vi "Exercise1.3-Accumulator_For.vi"() -> ()   [LabVIEW 2013]
panel:
  out "Array":i32[](array[numeric])
  out "Sum":i32
  in  "N":i32
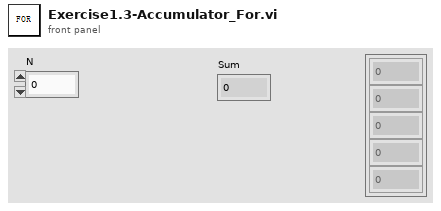
[diagram p1: front panel]
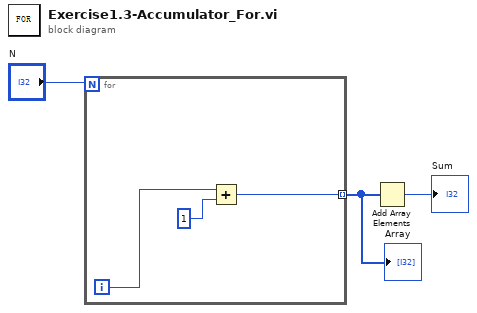
[diagram p0: block diagram]
diagram:
  n1 = for {
    N: "N" -> [_]
    tunnel: [w4] -> w2 mode=indexing
    i -> [w6]
    n2 = Add(x=w6, y=1) -> (x+y=w4:i32)
  }
  "Array" <- w2
  n3 = Add Array Elements(numeric array=w2) -> (sum=→"Sum":i32)
